vi "CreateUserEvents.vi"(8 "error in (no error)":errorcluster, 11 "UserEvents":T1) -> (0 "error out":errorcluster, 3 "UserEvents out":T1)   [LabVIEW 2022 SP3, in "IO.lvclass"]
uses:
  IO.lvclass
  Typedefs/UserEvents.ctl
  Typedefs/API Event Data.ctl
  Typedefs/API Task State.ctl
  Typedefs/Status Cluster.ctl
  Typedefs/ICP1-D0 Channel Names.ctl
  Typedefs/ICP2-DI Channel Names.ctl
  Typedefs/ICP2-DO Channel Names.ctl
  Typedefs/ICP1-AI Channel Names.ctl
  Typedefs/ICP1-AO Channel Names.ctl
  Typedefs/ICP2-AO Channel Names.ctl
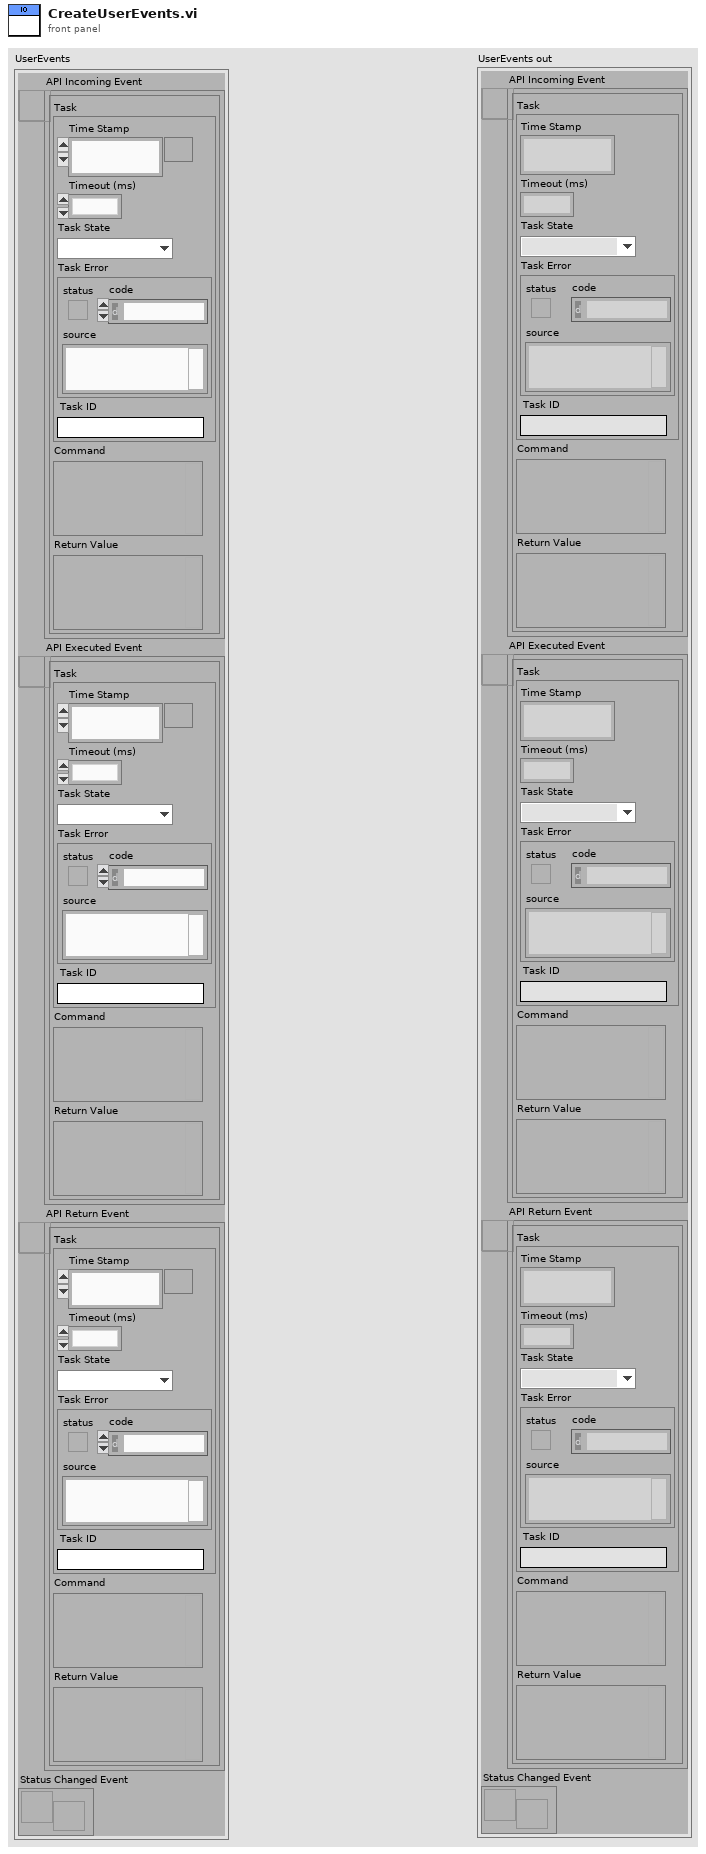
[diagram p1: front panel]
types:
  T1 = typedef "IO.lvclass/UserEvents.ctl" = cluster{"API Incoming Event":refnum<user-event>, "API Executed Event":refnum<user-event>, "API Return Event":refnum<user-event>, "Status Changed Event":refnum<user-event>}
  T2 = typedef "IO.lvclass/Status Cluster.ctl" = cluster{"Device Data":variant, "Ordered ICP1-DO Channels":T3[], "Ordered ICP2-DI Channels":T4[], "Ordered ICP2-DO Channels":T5[], "Ordered ICP1-AI Channels":T6[], "Ordered ICP1-AO Channels":T7[], "Ordered ICP2-AO Channels":T8[]}
  T3 = typedef "IO.lvclass/ICP1-D0 Channel Names.ctl" = enum16{"None", "Meniscus Pressure Reg PWR - R1", "Meniscus Pressure Reg PWR - R2", "Meniscus Pressure Reg PWR - R3", "Meniscus Pressure Reg PWR - R4", "Meniscus Pressure Reg PWR - R5", "Meniscus Pressure Reg PWR - R6", "Clear Stage Alarm", "Servo ON", "Purge Valve Open - R1", "Purge Valve Open - R2", "Purge Valve Open - R3", "Purge Valve Open - R4", "Purge Valve Open - R5", "Purge Valve Open - R6"}
  T4 = typedef "IO.lvclass/ICP2-DI Channel Names.ctl" = enum16{"None", "SW - Ink Valve - R1", "SW - Ink Valve - R2", "SW - Ink Valve - R3", "SW - Ink Valve - R4", "SW - Ink Valve - R5", "SW - Ink Valve - R6", "SW - COVER INPUT SIDE", "SW - COVER OUTPUT SIDE", "SW - Purge - R1", "SW - Purge - R2", "SW - Purge - R3", "SW - Purge - R4", "SW - Purge - R5", "SW - Purge - R6"}
  T5 = typedef "IO.lvclass/ICP2-DO Channel Names.ctl" = enum16{"None", "Meniscus Valve Open - R1", "Meniscus Valve Open - R2", "Meniscus Valve Open - R3", "Meniscus Valve Open - R4", "Meniscus Valve Open - R5", "Meniscus Valve Open - R6", "Ink Flow Valve Open - R1", "Ink Flow Valve Open - R2", "Ink Flow Valve Open - R3", "Ink Flow Valve Open - R4", "Ink Flow Valve Open - R5", "Ink Flow Valve Open - R6", "SW_LED - Ink Valve - R1", "SW_LED - Ink Valve - R2", "SW_LED - Ink Valve - R3", "Recirc Pump On - R1", "Recirc Pump On - R2", "Recirc Pump On - R3", "Recirc Pump On - R4", "Recirc Pump On - R5", "Recirc Pump On - R6", "SW_LED - Ink Valve - R4", "SW_LED - Ink Valve - R5", "SW_LED - Ink Valve - R6"}
  T6 = typedef "IO.lvclass/ICP1-AI Channel Names.ctl" = enum16{"None", "Meniscus Pressure Read - R1", "Meniscus Pressure Read - R2", "Meniscus Pressure Read - R3", "Meniscus Pressure Read - R4", "Meniscus Pressure Read - R5", "Meniscus Pressure Read - R6", "Meniscus Pressure Set - R1", "Meniscus Pressure Set - R2", "Meniscus Pressure Set - R3", "Meniscus Pressure Set - R4", "Meniscus Pressure Set - R5", "Meniscus Pressure Set - R6"}
  T7 = typedef "IO.lvclass/ICP1-AO Channel Names.ctl" = enum16{"None", "Meniscus Pressure Set - R1", "Meniscus Pressure Set - R2", "Meniscus Pressure Set - R3", "Meniscus Pressure Set - R4", "Meniscus Pressure Set - R5", "Meniscus Pressure Set - R6", "Meniscus Vac Pump Speed"}
  T8 = typedef "IO.lvclass/ICP2-AO Channel Names.ctl" = enum16{"None", "Recirc Pump Flow Set - R1", "Recirc Pump Flow Set - R2", "Recirc Pump Flow Set - R3", "Recirc Pump Flow Set - R4", "Recirc Pump Flow Set - R5", "Recirc Pump Flow Set - R6"}
  T9 = typedef "IO.lvclass/API Event Data.ctl" = cluster{"Task":cluster{"Time Stamp":timestamp, "Timeout (ms)":u32, "Task State":T10, "Task Error":errorcluster, "Task ID":string}, "Command":variant, "Return Value":variant}
  T10 = typedef "IO.lvclass/API Task State.ctl" = enum16{"Completed", "Errored", "Pending"}
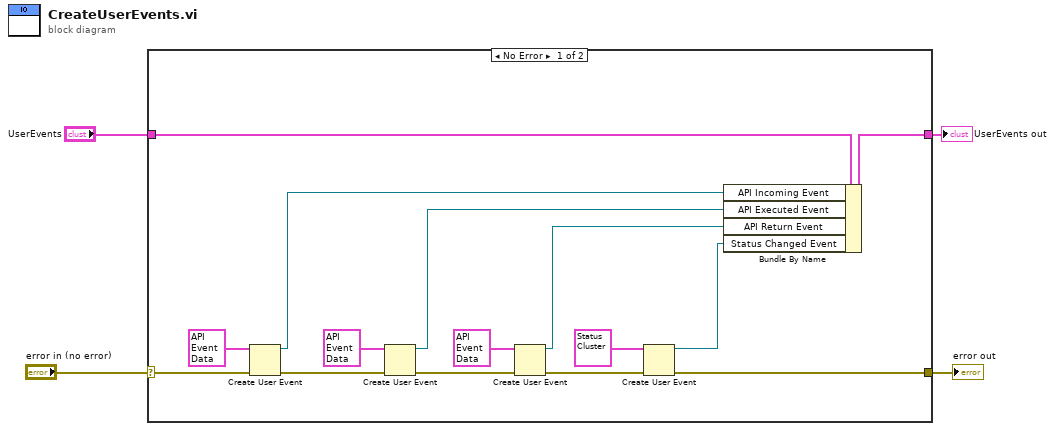
[diagram p0: block diagram]
diagram:
  n1 = case shown="No Error" "error in (no error)" {
    selector: "error in (no error)" -> [w15 w21]
    tunnel: [w6 w21] -> w3
    tunnel: "UserEvents" -> [w19 w20]
    tunnel: [w18 w20] -> w1
    frame No Error {
      n2 = Create User Event(user event datatype=T9 {"Task"={"Time Stamp"=timestamp(0 s since 1904-01-01), "Timeout (ms)"=0, "Task State"=enum."Completed", "Task Error"={"status"=FALSE, "code"=0, "source"=""}, "Task ID"=""}, "Command"=variant(enum16{"Event 1"} enum."Event 1"), "Return Value"=variant(string "")} ("API Event Data"), error in=w15) -> (user event=w16:refnum<user-event>, error out=w13:errorcluster)
      n3 = Create User Event(user event datatype=T9 {"Task"={"Time Stamp"=timestamp(0 s since 1904-01-01), "Timeout (ms)"=0, "Task State"=enum."Completed", "Task Error"={"status"=FALSE, "code"=0, "source"=""}, "Task ID"=""}, "Command"=variant(enum16{"Event 1"} enum."Event 1"), "Return Value"=variant(string "")} ("API Event Data"), error in=w13) -> (user event=w12:refnum<user-event>, error out=w10:errorcluster)
      n4 = Create User Event(user event datatype=T9 {"Task"={"Time Stamp"=timestamp(0 s since 1904-01-01), "Timeout (ms)"=0, "Task State"=enum."Completed", "Task Error"={"status"=FALSE, "code"=0, "source"=""}, "Task ID"=""}, "Command"=variant(enum16{"Event 1"} enum."Event 1"), "Return Value"=variant(string "")} ("API Event Data"), error in=w10) -> (user event=w9:refnum<user-event>, error out=w7:errorcluster)
      n5 = Create User Event(user event datatype=T2 {"Device Data"=variant, "Ordered ICP1-DO Channels"=[], "Ordered ICP2-DI Channels"=[], "Ordered ICP2-DO Channels"=[], "Ordered ICP1-AI Channels"=[], "Ordered ICP1-AO Channels"=[], "Ordered ICP2-AO Channels"=[]} ("Status"), error in=w7) -> (user event=w5:refnum<user-event>, error out=w6:errorcluster)
      n6 = Bundle By Name(cluster=w19, "API Incoming Event"=w16, "API Executed Event"=w12, "API Return Event"=w9, "Status Changed Event"=w5) -> (w18:T1)
    }
    frame Error {
    }
  }
  "error out" <- w3
  "UserEvents out" <- w1
